vi "Log Error.vi"(8 "error in (no error)":errorcluster, 11 "VI Name":string) -> (0 "error out":errorcluster)   [LabVIEW 2017]
doc: "This Vi is used to log the error details with time stamp. Every Month one file will be Created.\n\nOutput of the error cluster will be no error(clear error function not required).\n\nWire the input of VI name"
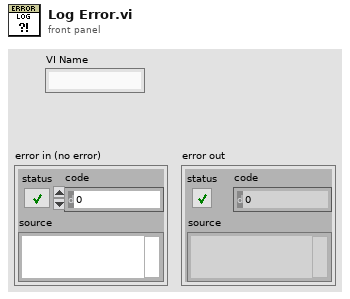
[diagram p1: front panel]
types:
  T1 = enum16{"open", "replace", "create", "open or create", "replace or create", "replace or create with confirmation"}
  T2 = typedef "Get Path - All Path Control.ctl" = cluster{"Source Code":path, "Exe":path, "data":path, "Dynamic VI's":path, "Plugable Drivers":path, "Error Logs":path, "Database":path, "Squence":path}
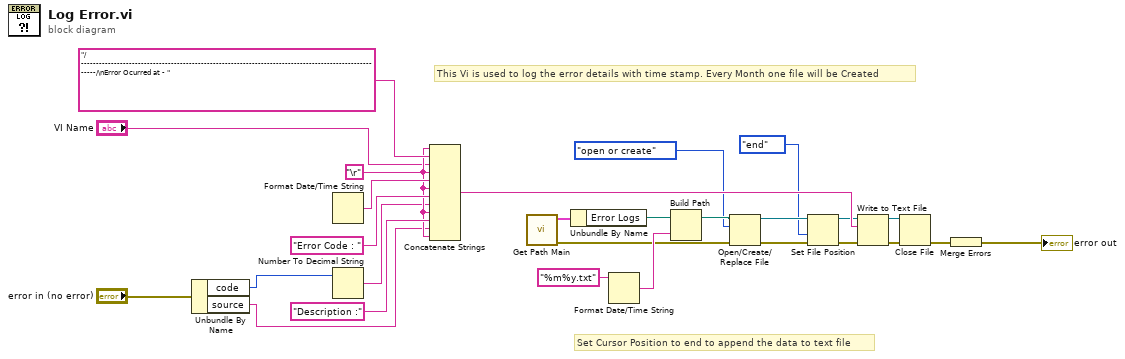
[diagram p0: block diagram]
diagram:
  w5 = "\r"
  # "Set Cursor Position to end to append the data to text file"
  # "This Vi is used to log the error details with time stamp. Every Month one file will be Created"
  n1 = Unbundle By Name("error in (no error)") -> ("code"=w23:i32, "source"=w3:string)
  n2 = Format Date/Time String() -> (date/time string=w26:string)  [unwired: 3 in]
  n3 = Number To Decimal String(number=w23) -> (decimal integer string=w4:string)  [unwired: 1 in]
  n4 = Concatenate Strings(w5, "/------------------------------------------------------------------------------------------------------/\nError Ocurred at - " ("string"), "VI Name", w5, w26, w5, "Error Code : " ("string"), w4, w5, "Description :" ("string"), w3, w5) -> (w17:string)
  n5 = call "Get Path Main.vi"() -> ("error out"=w16:errorcluster, "All Path"=w21:T2)  [unwired: 10 in]
  n6 = Unbundle By Name(w21) -> ("Error Logs"=w20:path)
  n7 = Format Date/Time String(time format string (%c)="%m%y.txt") -> (date/time string=w18:string)  [unwired: 2 in]
  n8 = Build Path(base path=w20, name or relative path=w18) -> (appended path=w15:path)
  n9 = Open/Create/Replace File(file path (use dialog)=w15, error in=w16, operation (0:open)=T1."open or create") -> (refnum out=w10:refnum<file>, error out=w8:errorcluster)  [unwired: 3 in, 1 out]
  n10 = Set File Position(refnum=w10, from (0:start)=enum16{"start", "end", "current"}."end", error in=w8) -> (refnum out=w9:refnum<file>, error out=w7:errorcluster)  [unwired: 1 in]
  n11 = Write to Text File(file (use dialog)=w9, text=w17, error in=w7) -> (refnum out=w12:refnum<file>, error out=w13:errorcluster)  [unwired: 1 in, 1 out]
  n12 = Close File(refnum=w12, error in=w13) -> (error out=w11:errorcluster)  [unwired: 1 out]
  n13 = Merge Errors(w11) -> (→"error out":errorcluster)
